vi "RSZVB Set Sweep Single.vi"(8 "error in (no error)":errorcluster {"code" format="%.0x"}, 9 "Single Sweep (1: Continuous Sweep)":i32(ring)=1 items=["Single Sweep", "Continuous Sweep"], 10 "Channel (1)":i32=1, 11 "VISA session":refnum<visa-resource-name>) -> (0 "error out":errorcluster {"code" format="%.0x"}, 3 "dup VISA session":refnum<visa-resource-name>)   [LabVIEW 2015]
doc: "This VI qualifies whether the analyzer measures in single sweep or in continuous sweep mode.\n\nRemote-control command(s):\nINITiate<Ch>:CONTinuous OFF | ON"
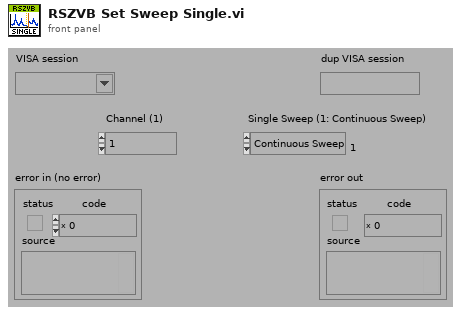
[diagram p1: front panel]
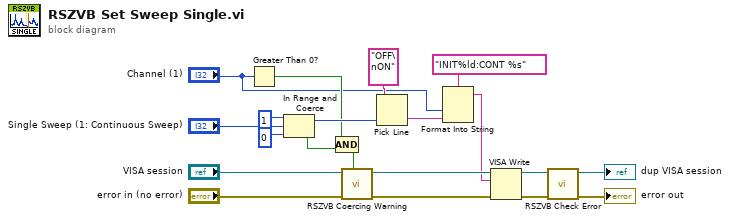
[diagram p0: block diagram]
diagram:
  n1 = Greater Than 0?(x="Channel (1)") -> (x > 0?=w9:bool)
  n2 = In Range and Coerce(upper limit=1, x="Single Sweep (1: Continuous Sweep)", lower limit=0) -> (coerced(x)=w17:i32, In Range?=w10:bool)
  n3 = Compound Arithmetic op=AND(w9, w10) -> (w8:bool)
  n4 = call "RSZVB Coercing Warning.vi"("In Range?"=w8, "error in (no error)"="error in (no error)", "VISA session"="VISA session") -> ("error out"=w14:errorcluster, "dup VISA session"=w15:refnum<visa-resource-name>)  [unwired: 7 in]
  n5 = Pick Line(multi-line string="OFF\nON", line index=w17) -> (output string=w11:string)  [unwired: 1 in]
  n6 = Format Into String(format string="INIT%ld:CONT %s", "Channel (1)", w11) -> (resulting string=w7:string)  [unwired: 2 in, 1 out]
  n7 = VISA Write(VISA resource name=w15, write buffer=w7, error in (no error)=w14) -> (VISA resource name out=w12:refnum<visa-resource-name>, error out=w13:errorcluster)  [unwired: 1 out]
  n8 = call "RSZVB Check Error.vi"("error in (no error)"=w13, "VISA session"=w12) -> ("error out"=→"error out":errorcluster, "dup VISA session"=→"dup VISA session":refnum<visa-resource-name>)  [unwired: 8 in]
